vi "Logging Example.vi"() -> ()   [LabVIEW 2016]
panel:
  in  "Data":dbl
  in  "Data 2":dbl
  out "System Time":string
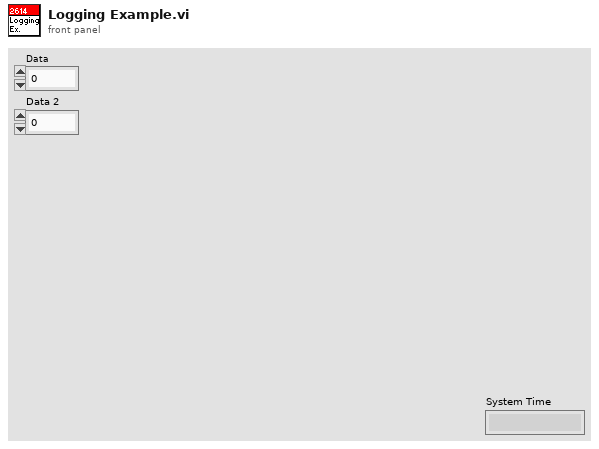
[diagram p1: front panel]
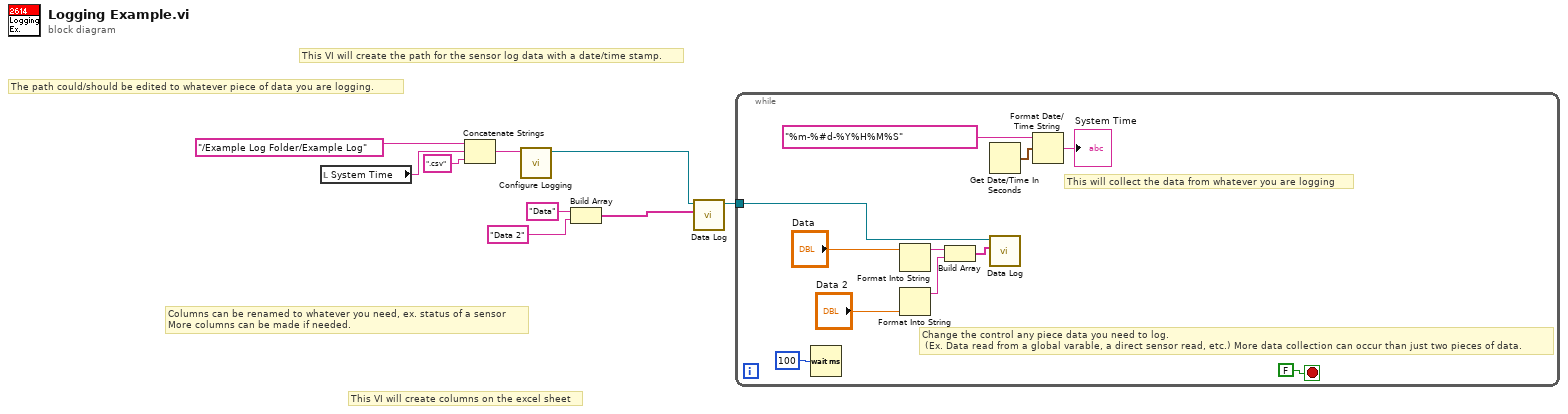
[diagram p0: block diagram]
diagram:
  # "Columns can be renamed to whatever you need, ex. status of a sensor\nMore columns can be made if needed."
  # "This VI will create columns on the excel sheet"
  # "This VI will create the path for the sensor log data with a date/time stamp."
  # "The path could/should be edited to whatever piece of data you are logging."
  n1 = local read "System Time"() -> (w7:string)
  n2 = Concatenate Strings("/Example Log Folder/Example Log" ("File Path/File Name"), w7, ".csv" ("string")) -> (w9:string)
  n3 = call "Configure Logging.vi"("File Path/File Name"=w9) -> ("refnum out"=w2:refnum<file>)  [unwired: 10 in]
  n4 = Build Array("Data" ("File Path/File Name"), "Data 2" ("File Path/File Name")) -> (w5:string[])
  n5 = call "Data Log.vi"("Data In"=w5, "File Reference In"=w2) -> ("File Reference Out"=w1:refnum<file>)  [unwired: 9 in]
  n6 = while {
    tunnel: w1 -> [w11]
    stop <- FALSE stop-if-true
    # "Change the control any piece data you need to log.\n (Ex. Data read from a global varable, a direct sensor read, etc.) More data collection can occur than just two pieces of data."
    # "This will collect the data from whatever you are logging"
    n7 = Wait (ms)(milliseconds to wait=u32 100) -> ()  [unwired: 1 out]
    n8 = Format Into String("Data") -> (resulting string=w12:string)  [unwired: 3 in, 1 out]
    n9 = Format Into String("Data 2") -> (resulting string=w15:string)  [unwired: 3 in, 1 out]
    n10 = Build Array(w12, w15) -> (w14:string[])
    n11 = Get Date/Time In Seconds() -> (seconds since 1Jan1904=w19:timestamp)
    n12 = call "Data Log.vi"("Data In"=w14, "File Reference In"=w11) -> ()  [unwired: 9 in, 1 out]
    n13 = Format Date/Time String(time format string (%c)="%m-%#d-%Y%H%M%S", seconds (now)=w19) -> (date/time string=→"System Time":string)  [unwired: 1 in]
  }
